vi "Read File (Complete).vi"(8 "error in (no error)":errorcluster, 11 "ConfigManager.Text in":refnum<class "ConfigManager.Text.lvclass">) -> (0 "error out":errorcluster, 2 "String":string, 3 "ConfigManager.Text out":refnum<class "ConfigManager.Text.lvclass">)   [LabVIEW 2013, in "CfgManager.Text.lvlib" / "ConfigManager.Text.lvclass"]
uses:
  ConfigManager.Text.lvclass
  ConfigManager.Text.lvclass/ConfigManager.Text.ctl
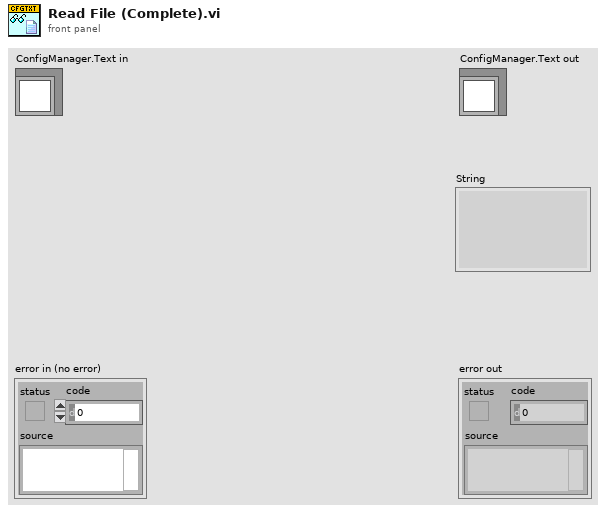
[diagram p1: front panel]
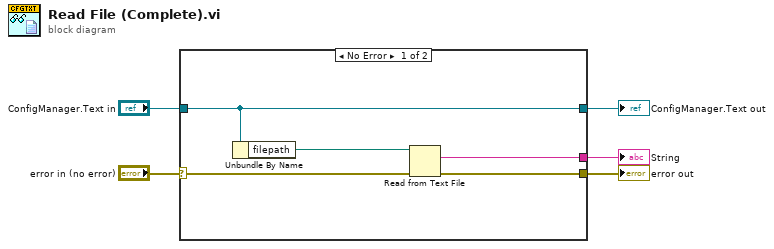
[diagram p0: block diagram]
diagram:
  n1 = case shown="No Error" "error in (no error)" {
    selector: "error in (no error)" -> [w7 w12]
    tunnel: [w6 w12] -> w4
    tunnel: [w9 w11] -> w2
    tunnel: "ConfigManager.Text in" -> [w9 w11]
    tunnel: [w8 _] -> w1
    frame No Error {
      n2 = Unbundle By Name(w9) -> ("filepath"=w10:path)
      n3 = Read from Text File(file (use dialog)=w10, error in=w7) -> (text=w8:string, error out=w6:errorcluster)  [unwired: 2 in, 2 out]
    }
    frame Error {
    }
  }
  "error out" <- w4
  "ConfigManager.Text out" <- w2
  "String" <- w1
